vi "Delete.vi"(8 "error in (no error)":errorcluster, 10 "Path":string, 11 "WebDAV in":refnum<class "WebDAV.lvclass">) -> (0 "error out":errorcluster, 3 "WebDAV out":refnum<class "WebDAV.lvclass">)   [LabVIEW 2015, in "RT Management.lvlib" / "WebDAV.lvclass"]
uses:
  WebDAV.lvclass
  WebDAV.lvclass/WebDAV.ctl
  Get Session.vi
  <vilib>/WebDAVClient/NI_WebDAV.lvlib
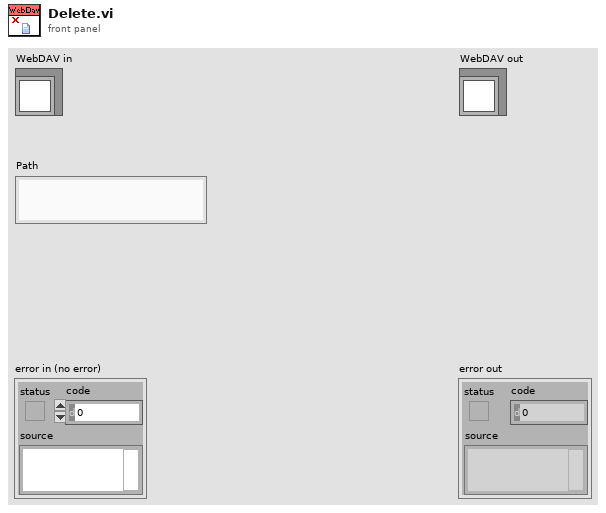
[diagram p1: front panel]
types:
  T1 = typedef "NI_WebDAV.lvlib/SessionHandle.ctl" = refnum<k1>
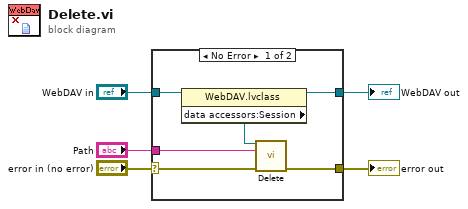
[diagram p0: block diagram]
diagram:
  n1 = case shown="No Error" "error in (no error)" {
    selector: "error in (no error)" -> [w6 w12]
    tunnel: "WebDAV in" -> [w11 w13]
    tunnel: "Path" -> [w10 _]
    tunnel: [w8 w12] -> w3
    tunnel: [w7 w13] -> w2
    frame No Error {
      n2 = property class="WebDAV.lvclass"(reference=w11) -> (reference out=w7:refnum<class "WebDAV.lvclass">, "data accessors:Session"=w9:T1)  [unwired: 1 in, 1 out]
      n3 = call <vilib>:"Delete.vi"("session handle"=w9, "relative uri"=w10, "error in (no error)"=w6) -> ("error out"=w8:errorcluster)  [unwired: 11 in, 1 out]
    }
    frame Error {
    }
  }
  "error out" <- w3
  "WebDAV out" <- w2
